vi "RNN - Read Params.vi"(0 "Parent Directory":path=path "C:/", 2 "Child Directory":path=path "misc/LabVIEW/FILES/TEST", 4 "identifier":string="test") -> (11 "files expected":i32=5, 13 "files found":i16=5, 14 "Paths":path[](array[path])=[path "C:/misc/LabVIEW/FILES/TEST/Wxh_test.psv", path "C:/misc/LabVIEW/FILES/TEST/Whh_test.psv", path "C:/misc/LabVIEW/FILES/TEST/bh_test.psv", path "C:/misc/LabVIEW/FILES/TEST/Why_test.psv", path "C:/misc/LabVIEW/FILES/TEST/by_test.psv"], 16 "params_":T2={"Wxh"=[[0.578129, 2.57297278, 0.17801602], [-2.46959, 0.02723142, 2.44961435]], "Whh"=[[-1.19960012, 0.76255511], [-0.03543363, -0.47610148]], "bh"=[[0.93535066], [-1.98598701]], "Why"=[[-0.85861611, 0.76469236], [-1.37899876, 0.188036], [-0.13091207, -0.33398775]], "by"=[[-0.728417], [-0.44032], [-0.88448186]]}, 19 "Params Loaded?":bool)   [LabVIEW 2014]
uses:
  <vilib>/Analysis/Matrix/Datatypes/RealMatrix.ctl
  <vilib>/Analysis/Matrix/Numeric/Conversions/Array To Matrix - RA2.vi
  <vilib>/Analysis/Matrix/NI_Matrix.lvlib
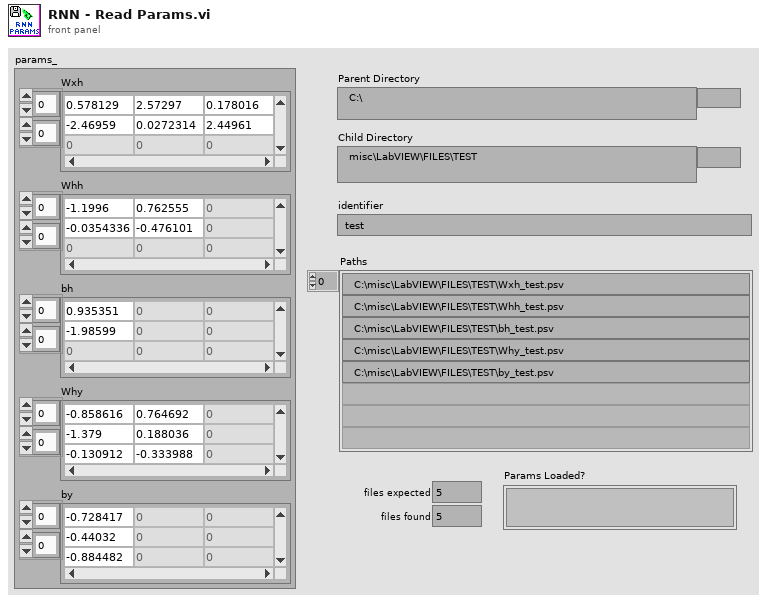
[diagram p1: front panel]
types:
  T1 = typedef "NI_Matrix.lvlib/RealMatrix.ctl" = dbl[][]
  T2 = cluster{"Wxh":T1, "Whh":T1, "bh":T1, "Why":T1, "by":T1}
  T3 = cluster{"Real Matrix":T1, "Real Matrix":T1, "Real Matrix":T1, "Real Matrix":T1, "Real Matrix":T1}
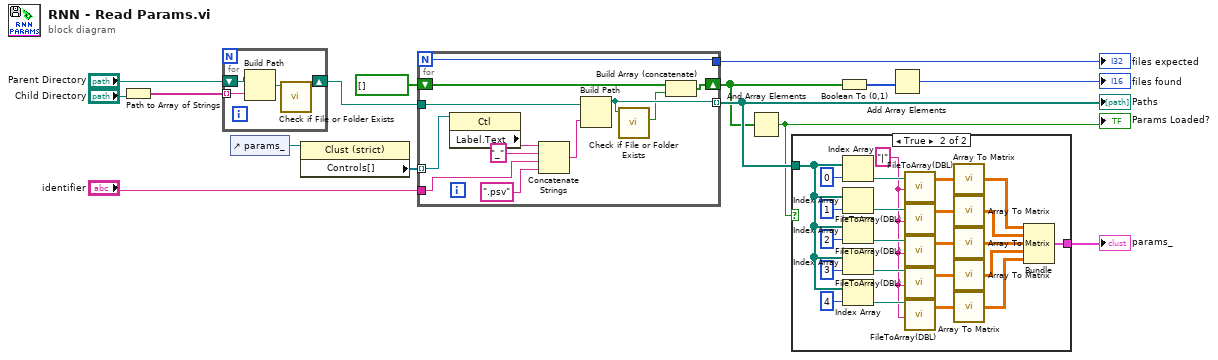
[diagram p0: block diagram]
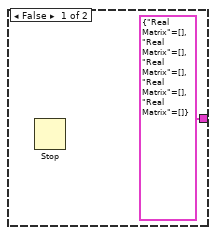
[diagram p2: hidden frame]
diagram:
  n1 = Path to Array of Strings(0:"Child Directory") -> (2:w11:string[])  [unwired: 1 out]
  n2 = for {
    tunnel: w11 -> [w18] mode=indexing
    shift-right: [w16] -> w9
    shift-left: "Parent Directory" -> [w19]
    n3 = Build Path(base path=w19, name or relative path=w18) -> (appended path=w17:path)
    n4 = call <vilib>:"Check if File or Folder Exists.vi"("path"=w17) -> ("dup path"=w16:path)  [unwired: 8 in, 2 out]
  }
  n5 = control-ref of="params_"() -> (w13:refnum<vi>)
  n6 = property class="Clust (strict)"(reference=w13) -> ("Controls[]"=w14:refnum<vi>[])  [unwired: 1 in, 2 out]
  n7 = for {
    N -> [w20]
    tunnel: w14 -> [w28] mode=indexing
    tunnel: w9 -> [w31]
    tunnel: [w24] -> w7 mode=indexing
    tunnel: "identifier" -> [w25]
    shift-right: [w22] -> w5
    shift-left: bool[] [] -> [w21]
    tunnel: [w20] -> w2
    n8 = property class="Ctl"(reference=w28) -> ("Label.Text"=w29:string)  [unwired: 1 in, 2 out]
    n9 = Concatenate Strings(w29, "_" ("string"), w25, ".psv" ("string")) -> (w30:string)
    n10 = Build Path(base path=w31, name or relative path=w30) -> (appended path=w24:path)
    n11 = call <vilib>:"Check if File or Folder Exists.vi"("path"=w24) -> ("file or folder exists?"=w23:bool)  [unwired: 8 in, 2 out]
    n12 = Build Array (concatenate)(w21, w23) -> (w22:bool[])
  }
  "Paths" <- w7
  "files expected" <- w2
  n13 = And Array Elements(Boolean array=w5) -> (logical AND=w1:bool)
  "Params Loaded?" <- w1
  n14 = case shown="True" w1 {
    tunnel: [T3 {"Real Matrix"=[], "Real Matrix"=[], "Real Matrix"=[], "Real Matrix"=[], "Real Matrix"=[]} w40] -> w8
    tunnel: w7 -> [_ w33]
    frame False {
      n15 = Stop() -> ()  [unwired: 1 in]
    }
    frame True {
      w34 = "|" ("string")
      n16 = Index Array(array=w33, index=0) -> (element=w39:path)
      n17 = Index Array(array=w33, index=1) -> (element=w38:path)
      n18 = Index Array(array=w33, index=2) -> (element=w37:path)
      n19 = Index Array(array=w33, index=3) -> (element=w36:path)
      n20 = Index Array(array=w33, index=4) -> (element=w35:path)
      n21 = call "FileToArray(DBL).vi"("path"=w39, "delimiter"=w34) -> ("data"=w50:dbl[][])  [unwired: 15 in, 2 out]
      n22 = call "FileToArray(DBL).vi"("path"=w38, "delimiter"=w34) -> ("data"=w49:dbl[][])  [unwired: 15 in, 2 out]
      n23 = call "FileToArray(DBL).vi"("path"=w37, "delimiter"=w34) -> ("data"=w48:dbl[][])  [unwired: 15 in, 2 out]
      n24 = call "FileToArray(DBL).vi"("path"=w36, "delimiter"=w34) -> ("data"=w47:dbl[][])  [unwired: 15 in, 2 out]
      n25 = call "FileToArray(DBL).vi"("path"=w35, "delimiter"=w34) -> ("data"=w46:dbl[][])  [unwired: 15 in, 2 out]
      n26 = call-poly <vilib>:"Array To Matrix.vi"("Real 2D Array"=w50) -> ("Real Matrix"=w45:T1)
      n27 = call-poly <vilib>:"Array To Matrix.vi"("Real 2D Array"=w49) -> ("Real Matrix"=w44:T1)
      n28 = call-poly <vilib>:"Array To Matrix.vi"("Real 2D Array"=w48) -> ("Real Matrix"=w43:T1)
      n29 = call-poly <vilib>:"Array To Matrix.vi"("Real 2D Array"=w47) -> ("Real Matrix"=w42:T1)
      n30 = call-poly <vilib>:"Array To Matrix.vi"("Real 2D Array"=w46) -> ("Real Matrix"=w41:T1)
      n31 = Bundle("Real Matrix"=w45, "Real Matrix"=w44, "Real Matrix"=w43, "Real Matrix"=w42, "Real Matrix"=w41) -> (w40:T3)  [unwired: 1 in]
    }
  }
  "params_" <- w8
  n32 = Boolean To (0,1)(Boolean=w5) -> (0, 1=w4:i16[])
  n33 = Add Array Elements(numeric array=w4) -> (sum=→"files found":i16)
